vi "Expt10.vi"() -> ()   [LabVIEW 2020]
panel:
  out "current time":timestamp
  out "den":dbl
  out "num":dbl
  out "Monthly Payment 2":dbl
  in  "Months 2":dbl
  in  "Interest Rate 2":dbl
  in  "Loan Amount":dbl
  out "Monthly Payment":dbl
  in  "Loan":dbl
  in  "Months":dbl
  in  "Interest Rate":dbl
  # "1)"
  # "2)"
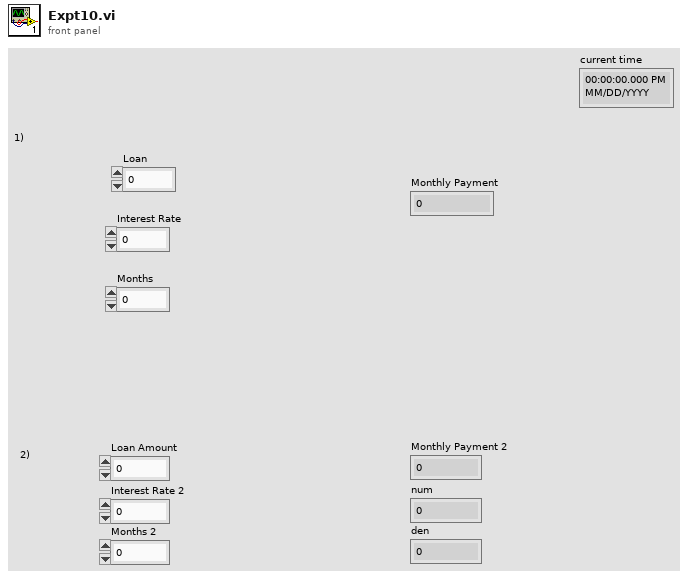
[diagram p1: front panel]
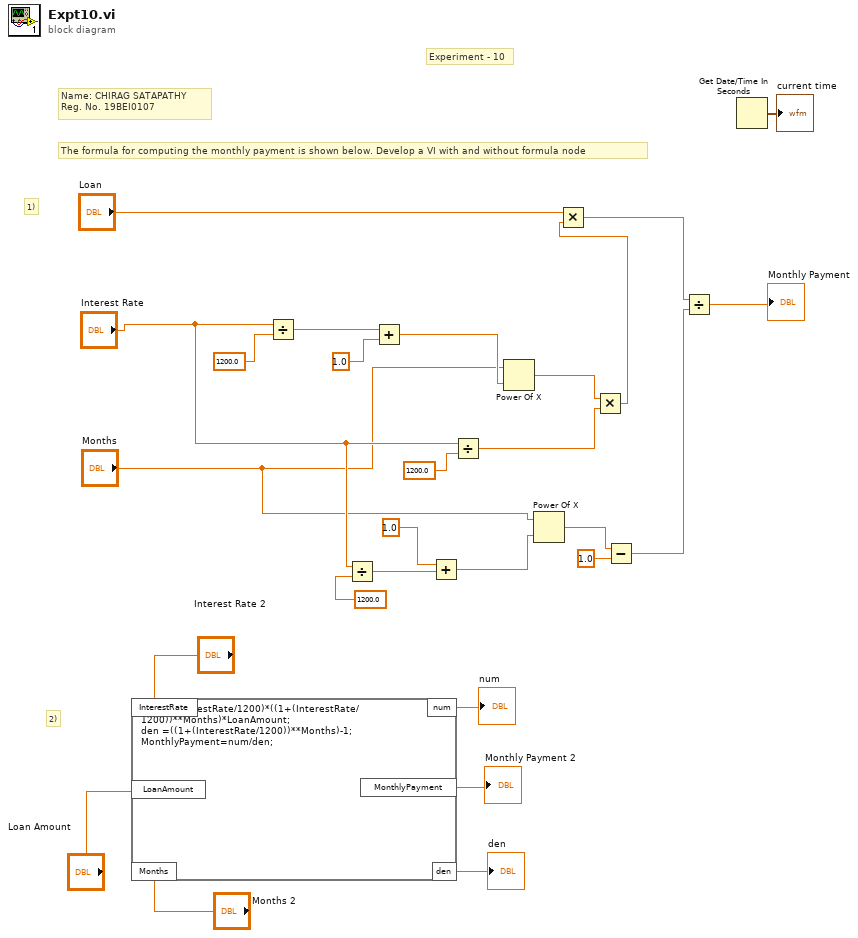
[diagram p0: block diagram]
diagram:
  # "1)"
  # "2)"
  # "Experiment - 10"
  # "Name: CHIRAG SATAPATHY\nReg. No. 19BEI0107"
  # "The formula for computing the monthly payment is shown below. Develop a VI with and without formula node"
  n1 = formula code="num=(InterestRate/1200)*((1+(InterestRate/1200))**Months)*LoanAmount;\nden =((1+(InterestRate/1200))**Months)-1;\nMonthlyPayment=num/den;"("LoanAmount"="Loan Amount", "InterestRate"="Interest Rate 2", "Months"="Months 2") -> ("MonthlyPayment"=→"Monthly Payment 2":dbl, "num"=→"num":dbl, "den"=→"den":dbl)
  n2 = Divide(x="Interest Rate", y=1200.0) -> (x/y=w25:dbl)
  n3 = Divide(x="Interest Rate", y=1200.0) -> (x/y=w14:dbl)
  n4 = Add(x=w25, y=1.0) -> (x+y=w23:dbl)
  n5 = Add(x=1.0, y=w14) -> (x+y=w11:dbl)
  n6 = Divide(x="Interest Rate", y=1200.0) -> (x/y=w21:dbl)
  n7 = Power Of X(1:w23, 2:"Months") -> (0:w20:dbl)
  n8 = Power Of X(1:w11, 2:"Months") -> (0:w16:dbl)
  n9 = Multiply(x=w20, y=w21) -> (x*y=w19:dbl)
  n10 = Multiply(x="Loan", y=w19) -> (x*y=w18:dbl)
  n11 = Subtract(x=w16, y=1.0) -> (x-y=w17:dbl)
  n12 = Divide(x=w18, y=w17) -> (x/y=→"Monthly Payment":dbl)
  n13 = Get Date/Time In Seconds() -> (seconds since 1Jan1904=→"current time":timestamp)
